vi "Convert from String.vi"(8 "error in":errorcluster, 11 "KA string":string="DB_Query=\"Select\" Connection=\"c:\\Temp\" ") -> (0 "error out":errorcluster, 3 "keyed array":T1)   [LabVIEW 2012, in "TLB` Template.lvlib" / "Tools_KeyedArray.lvlib"]
uses:
  Tools_KeyedArray.lvlib
  KeyedArray.ctl
  Map String.vi
  String/Get Case Matching.vi
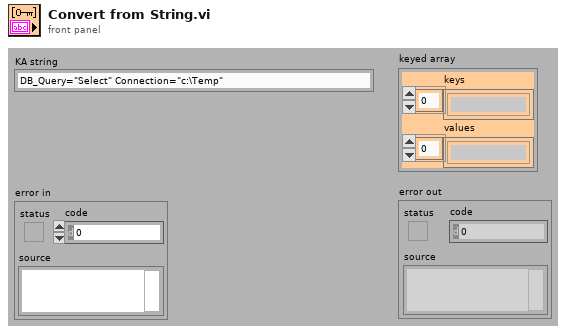
[diagram p1: front panel]
types:
  T1 = typedef "TLB` Template.lvlib/Tools_KeyedArray.lvlib/KeyedArray.ctl" = cluster{"keys":string[], "values":string[]}
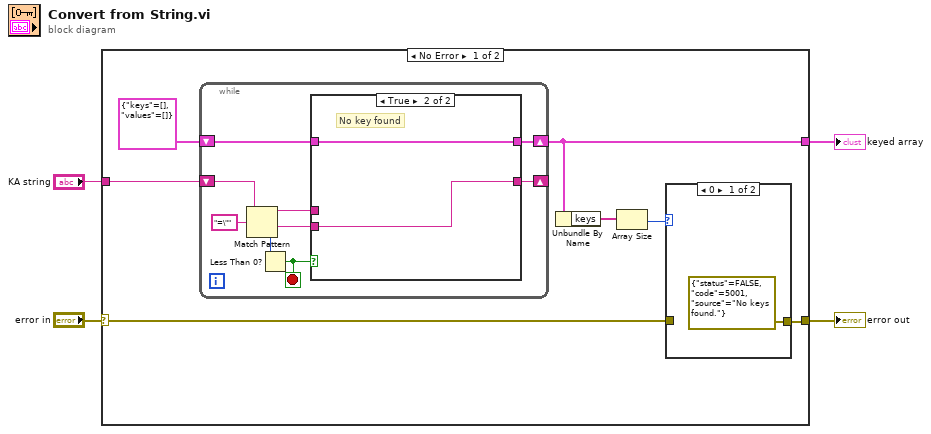
[diagram p0: block diagram]
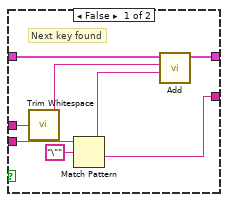
[diagram p3: hidden frame]
diagram:
  n1 = case shown="No Error" "error in" {
    selector: "error in" -> [w5 w33]
    tunnel: [w8 w33] -> w3
    tunnel: [w7 _] -> w2
    tunnel: "KA string" -> [w6 _]
    frame No Error {
      n2 = while {
        shift-right: [w14] -> _
        shift-left: w6 -> [w22]
        shift-right: [w16] -> w7
        shift-left: T1 {"keys"=[], "values"=[]} ("keyed array") -> [w17]
        stop <- w19 stop-if-true
        n3 = Match Pattern(string=w22, regular expression="=\"") -> (before substring=w18:string, after substring=w15:string, offset past match=w20:i32)  [unwired: 2 out]
        n4 = Less Than 0?(x=w20) -> (x < 0?=w19:bool)
        n5 = case shown="True" w19 {
          tunnel: w18 -> [w30 _]
          tunnel: w17 -> [w29 w32]
          tunnel: [w28 w32] -> w16
          tunnel: w15 -> [w26 w31]
          tunnel: [w23 w31] -> w14
          frame False {
            # "Next key found"
            n6 = call <vilib>:"Trim Whitespace.vi"("string"=w30) -> ("trimmed string"=w27:string)  [unwired: 1 in]
            n7 = Match Pattern(string=w26, regular expression="\"") -> (before substring=w24:string, after substring=w23:string)  [unwired: 3 out]
            n8 = call "Add.vi"("value"=w24, "key"=w27, "array in"=w29) -> ("array out"=w28:T1)  [unwired: 1 in, 3 out]
          }
          frame True {
            # "No key found"
          }
        }
      }
      n9 = Unbundle By Name(w7) -> ("keys"=w10:string[])
      n10 = Array Size(array=w10) -> (size(s)=w9:i32)
      n11 = case shown="0" w9 {
        tunnel: [errorcluster {"status"=FALSE, "code"=5001, "source"="No keys found."} ("error IO") w13] -> w8
        tunnel: w5 -> [_ w13]
        frame 0 {
        }
        frame 1, Default {
        }
      }
    }
    frame Error {
    }
  }
  "error out" <- w3
  "keyed array" <- w2
